vi "Update Step Go To Action If Necessary.vi"(6 "Action case (T/F)":bool, 7 "TreeControl in":refnum<vi>, 9 "Step Update Map in":T1(c390), 10 "Step Number":i32, 11 "Step Settings in":T2) -> (0 "Action removed":bool, 1 "Step Update Map out":T1(c390), 2 "Action updated":bool, 3 "Step Settings out":T2)   [LabVIEW 2020, in "Output Sequencer.lvlib" / "Settings UI.lvclass"]
uses:
  Settings UI.lvclass
  Types/Step Settings.ctl
  Types/Tree Index Enum.ctl
  Globals/Global Tree Data.vi
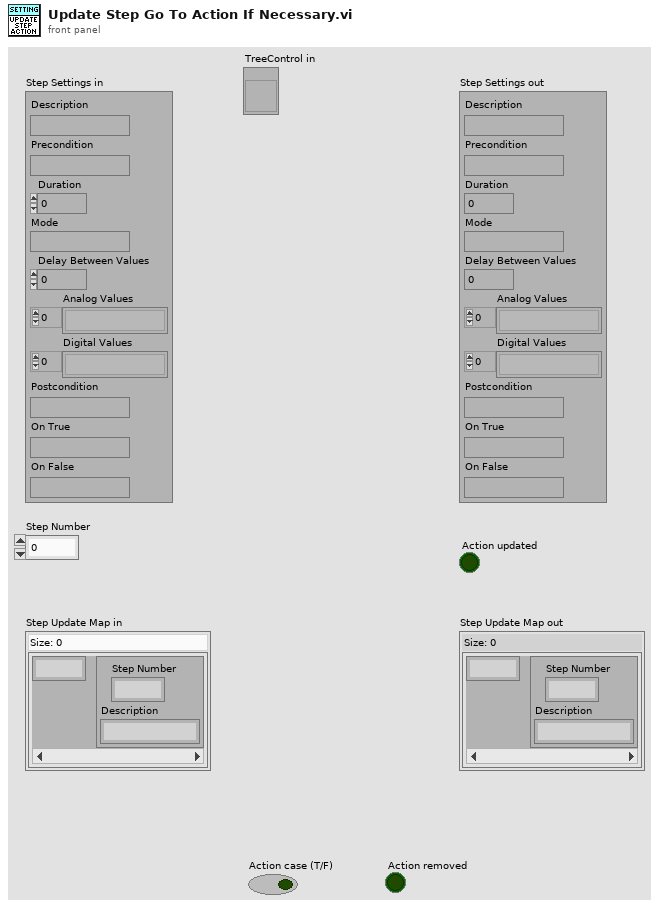
[diagram p1: front panel]
types:
  T1 = map{i32, cluster{"Step Number":i32, "Description":string}}
  T2 = typedef "Output Sequencer.lvlib/Settings UI.lvclass/Step Settings.ctl" = cluster{"Description":string, "Precondition":string, "Duration":dbl, "Mode":string, "Delay Between Values":dbl, "Analog Values":string[], "Digital Values":string[], "Postcondition":string, "On True":string, "On False":string}
  T3 = typedef "Output Sequencer.lvlib/Settings UI.lvclass/Tree Index Enum.ctl" = enum16{"General Settings", "Num Steps", "Num Analog", "Num Digital", "Show Confirmation", "Interp Priority", "Adv Timing", "Enable Conditions", "Seq Execution", "Reset Test Start", "Only When Test", "Delay After Test", "Start condition", "Re-triggering", "Stop condition", "Stop After Cycles", "Stop Values", "Default Values", "Default Analog", "Default Digital", "Steps", "Step #", "Description", "Precondition", "Duration", "Mode", "Delay Between Vals", "Analog Values", "Digital Values", "Postcondition", "On True", "On False"}
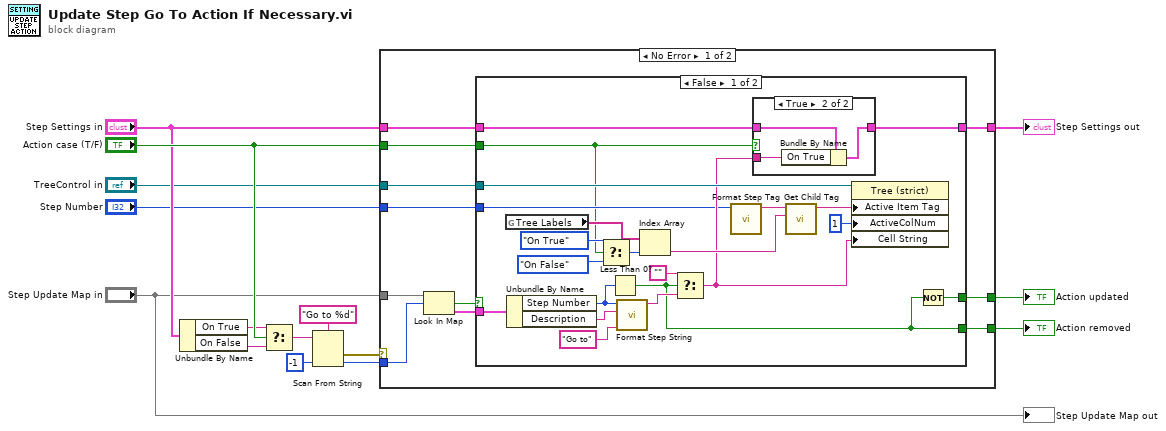
[diagram p0: block diagram]
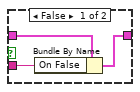
[diagram p2: hidden frame]
diagram:
  n1 = Unbundle By Name("Step Settings in") -> ("On True"=w13:string, "On False"=w14:string)
  n2 = Select(t=w13, s="Action case (T/F)", f=w14) -> (s? t:f=w3:string)
  n3 = Scan From String(format string="Go to %d", input string=w3, default 1=-1 ("default value 1")) -> (error out=w9:errorcluster, output 1=w8:i32)  [unwired: 2 in, 2 out]
  n4 = case shown="No Error" w9 {
    tunnel: "Step Settings in" -> [w26 w56]
    tunnel: [w25 w56] -> w6
    tunnel: "Step Number" -> [w24 _]
    tunnel: "TreeControl in" -> [w23 _]
    tunnel: "Step Update Map in" -> [w22 _]
    tunnel: w8 -> [w21 _]
    tunnel: [w18 _] -> w10
    tunnel: "Action case (T/F)" -> [w17 _]
    tunnel: [w16 _] -> w1
    frame No Error {
      n5 = Look In Map(map=w22, key=w21) -> (key not found?=w19:bool, value=w20:cluster{"Step Number":i32, "Description":string})  [unwired: 1 in]
      n6 = case shown="False" w19 {
        tunnel: w20 -> [w40 _]
        tunnel: w26 -> [w48 w55]
        tunnel: [w47 w55] -> w25
        tunnel: w24 -> [w37 _]
        tunnel: w23 -> [w43 _]
        tunnel: [w28 _] -> w18
        tunnel: w17 -> [w29 _]
        tunnel: [w27 _] -> w16
        frame False {
          n7 = global read "Global Tree Data.vi" "Tree Labels"() -> (w46:string[])
          n8 = Unbundle By Name(w40) -> ("Step Number"=w36:i32, "Description"=w33:string)
          n9 = Select(t=Tree_Index_Enum."On True" ("Tree Index Enum"), s=w29, f=Tree_Index_Enum."On False" ("Tree Index Enum")) -> (s? t:f=w30:T3)
          n10 = Less Than 0?(x=w36) -> (x < 0?=w28:bool)
          n11 = call "Format Step String.vi"("Initial string (default: \"Step\")"="Go to" ("Initial string (default: \"Step\")"), "Description"=w33, "Step Number"=w36) -> ("Step String out"=w34:string)  [unwired: 8 in]
          n12 = Index Array(array=w46, index=w30) -> (element=w44:string)
          n13 = Select(t="", s=w28, f=w34) -> (s? t:f=w38:string)
          n14 = call "Format Step Tag.vi"("Step Number"=w37) -> ("Tag"=w45:string)  [unwired: 10 in]
          n15 = case shown="True" w29 {
            tunnel: w48 -> [w50 w54]
            tunnel: [w51 w53] -> w47
            tunnel: w38 -> [w49 w52]
            frame False {
              n16 = Bundle By Name(cluster=w50, "On False"=w49) -> (w51:T2)
            }
            frame True {
              n17 = Bundle By Name(cluster=w54, "On True"=w52) -> (w53:T2)
            }
          }
          n18 = call "Get Child Tag.vi"("Child label"=w44, "Parent tag"=w45) -> ("Child tag"=w42:string)  [unwired: 9 in]
          n19 = property class="Tree (strict)"(reference=w43, "Active Item Tag"=w42, "ActiveColNum"=1 ("Active Cell:Active Column Number"), "Cell String"=w38) -> ()  [unwired: 1 in, 2 out]
          n20 = Not(x=w28) -> (.not. x?=w27:bool)
        }
        frame True {
        }
      }
    }
    frame Error {
    }
  }
  "Action removed" <- w10
  "Step Settings out" <- w6
  "Action updated" <- w1
  "Step Update Map out" <- "Step Update Map in"
